vi "Easy2Acquire.IDevice.Acquire.vi"(0 "IDeviceIn":refnum<k7>, 1 "IAnalogInput":refnum<k7>[](array[refnum]), 3 "DigitalInput":refnum<k7>[](array[refnum]), 4 "MotionInput":refnum<k7>[](array[refnum]), 5 "error in (no error)":errorcluster, 6 "stopcapture":refnum<vi>, 7 "AnalgoChart":refnum<vi>, 9 "endprogram":refnum<vi>, 10 "3DRef":refnum<vi>, 11 "DigitalChart":refnum<vi>, 12 "3D Picture":refnum<vi>, 13 "MotionChart":refnum<vi>) -> (14 "AnalogBuffer":dbl[][](array[numeric]), 17 "MotionBuffer":dbl[][][](array[numeric]), 18 "Euler":dbl[][][](array[numeric]), 19 "error out":errorcluster)   [LabVIEW 2017]
panel:
  out "DigitalFrequency":dbl[](array[numeric])
  out "MotionFrequency":dbl[](array[numeric])
  out "DigitalBuffer":i32[][](array[numeric])
  out "ActualFrequency":dbl[](array[numeric])
  in  "stop":bool
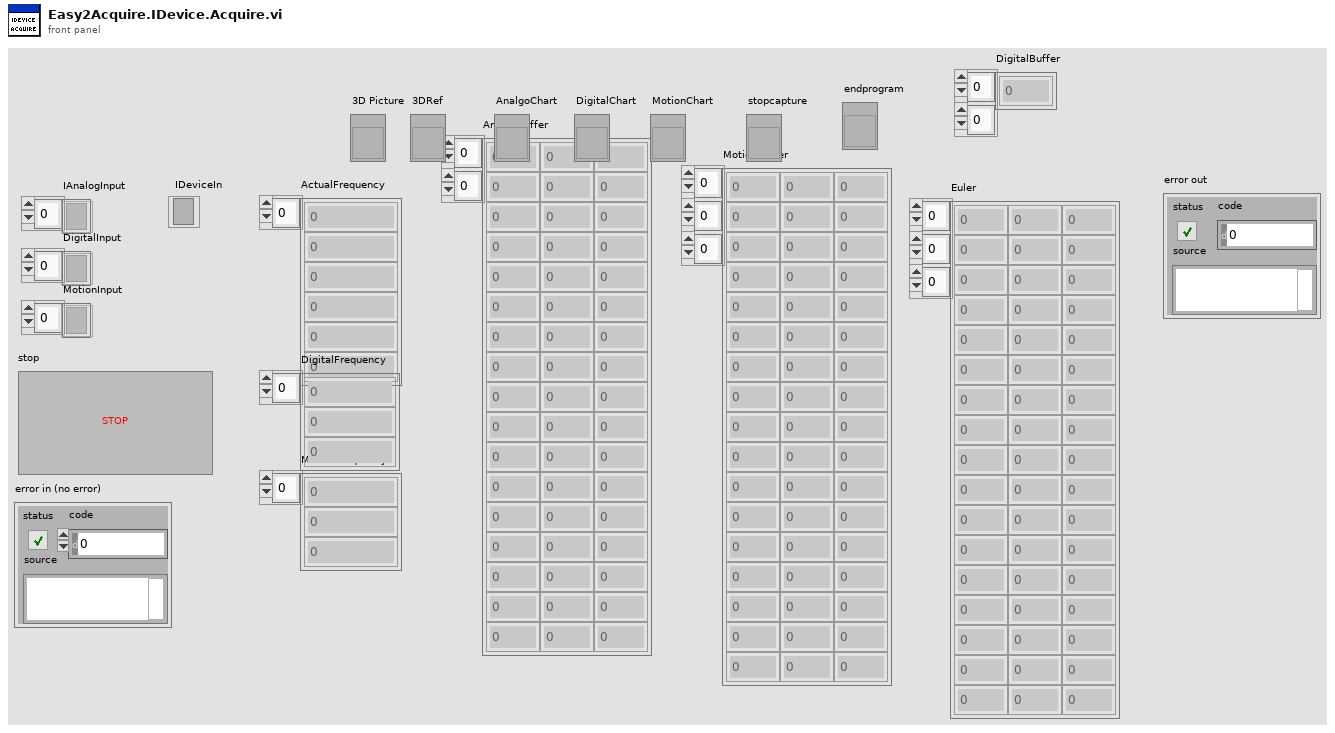
[diagram p1: front panel]
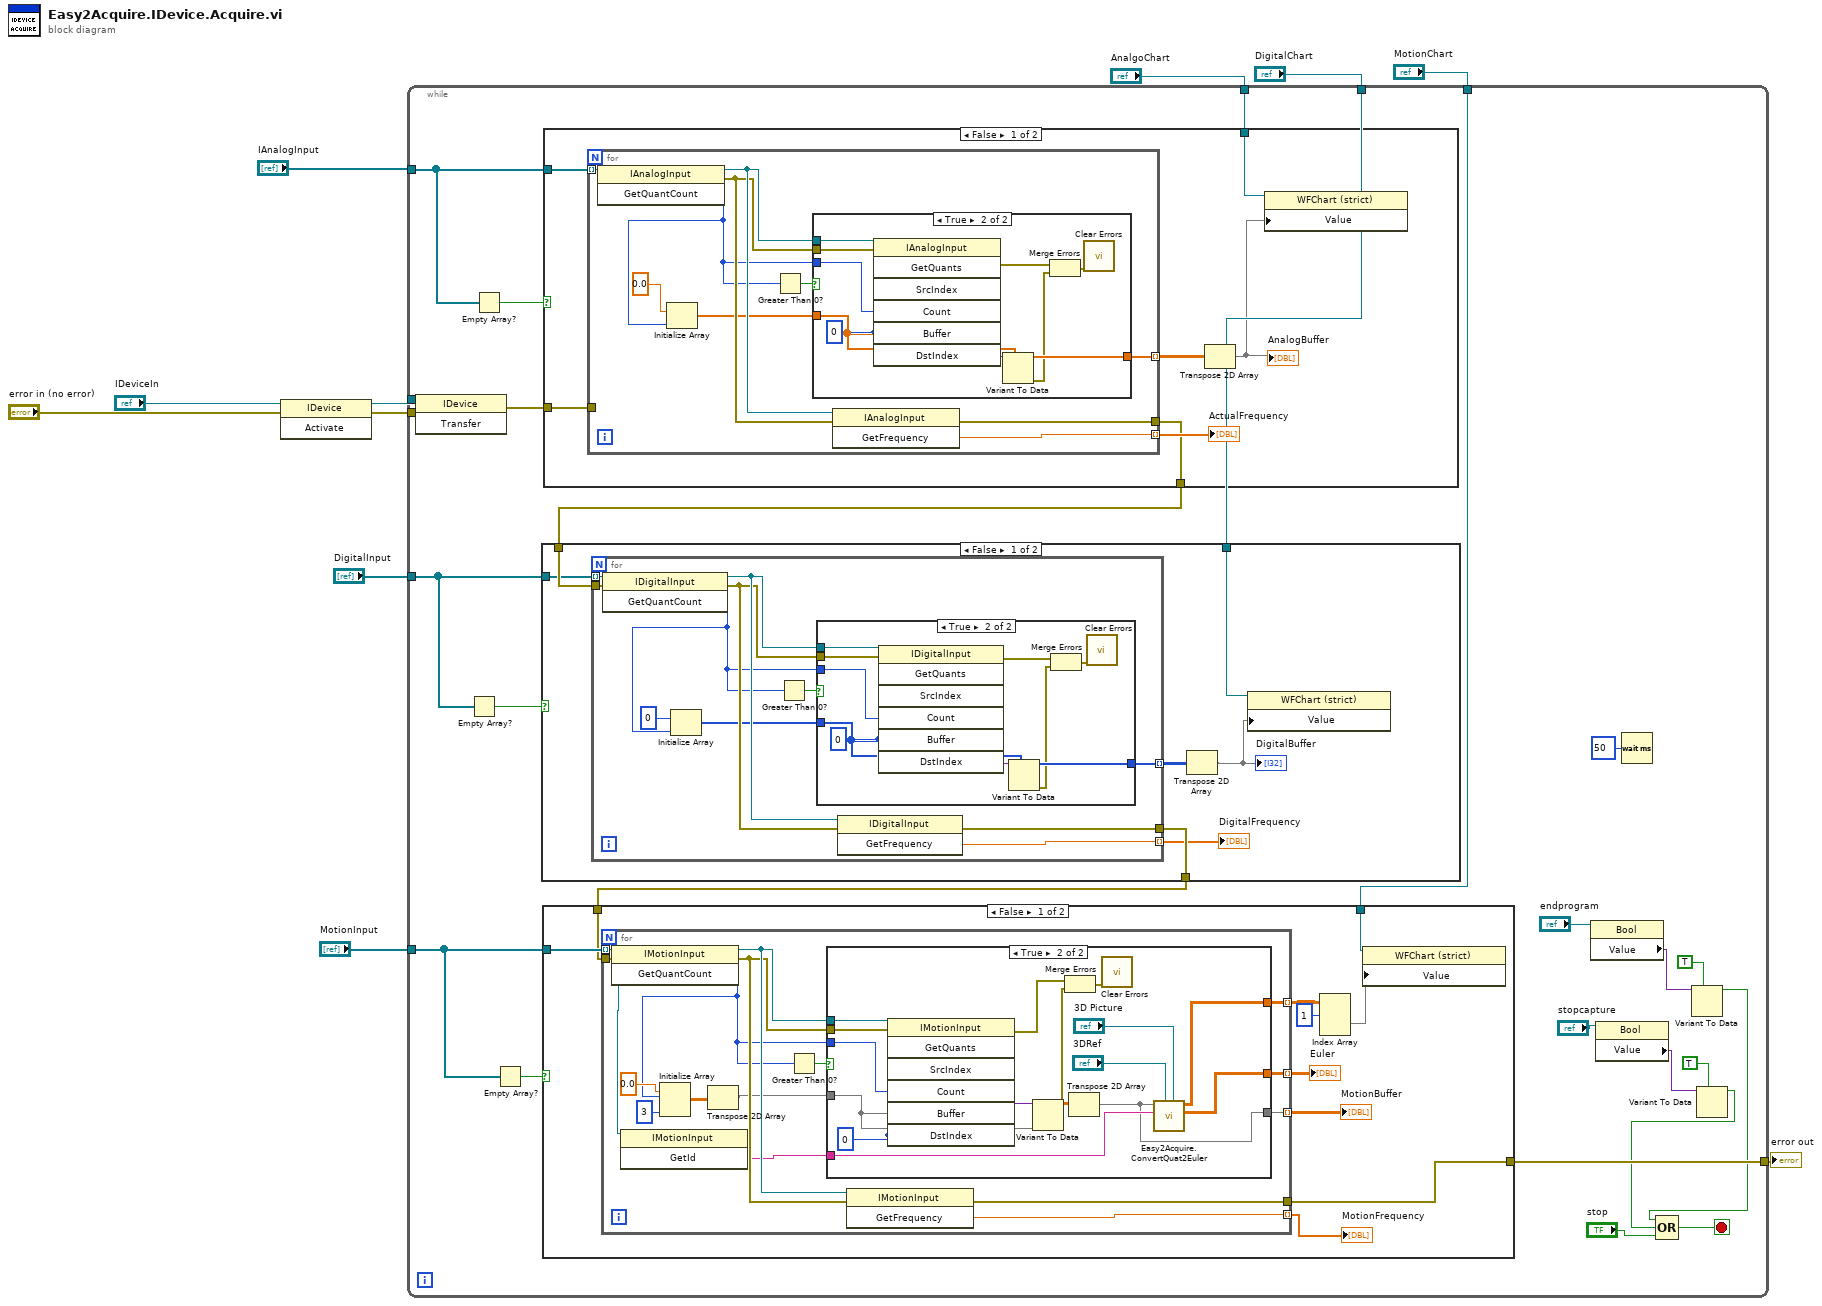
[diagram p0: block diagram]
diagram:
  n1 = invoke class="IDevice" method="Activate"(reference="IDeviceIn", error in="error in (no error)") -> (reference out=w10:refnum<k7>, error out=w9:errorcluster)  [unwired: 1 in, 1 out]
  n2 = while {
    tunnel: "IAnalogInput" -> [w22]
    tunnel: w9 -> [w37]
    tunnel: w10 -> [w36]
    tunnel: "DigitalInput" -> [w20]
    tunnel: "MotionInput" -> [w17]
    tunnel: [w31] -> w4
    tunnel: "AnalgoChart" -> [w30]
    tunnel: "DigitalChart" -> [w23]
    tunnel: "MotionChart" -> [w16]
    stop <- w27 stop-if-true
    n3 = invoke class="IDevice" method="Transfer"(reference=w36, error in=w37) -> (error out=w34:errorcluster)  [unwired: 1 in, 2 out]
    n4 = Empty Array?(array=w20) -> (empty?=w19:bool)
    n5 = Empty Array?(array=w22) -> (empty?=w21:bool)
    n6 = Empty Array?(array=w17) -> (empty?=w18:bool)
    n7 = case shown="False" w21 {
      tunnel: w22 -> [w116 _]
      tunnel: w34 -> [w114 w137]
      tunnel: [w113 w137] -> w33
      tunnel: w30 -> [w112 _]
      frame False {
        n8 = for {
          tunnel: w116 -> [w126] mode=indexing
          tunnel: [w124] -> w115 mode=indexing
          tunnel: [w118] -> w111 mode=indexing
          tunnel: w114 -> [_]
          tunnel: [w117] -> w113
          n9 = invoke class="IAnalogInput" method="GetQuantCount"(reference=w126) -> (reference out=w123:refnum<k7>, error out=w122:errorcluster, "GetQuantCount"=w120:i32)  [unwired: 2 in]
          n10 = Initialize Array(0.0, w120) -> (w121:dbl[])
          n11 = Greater Than 0?(x=w120) -> (x > 0?=w125:bool)
          n12 = case shown="True" w125 {
            tunnel: w123 -> [_ w136]
            tunnel: w120 -> [_ w135]
            tunnel: w122 -> [_ w133]
            tunnel: w121 -> [_ w131]
            tunnel: [_ w130] -> w118
            frame False {
            }
            frame True {
              w134 = 0 ("SrcIndex")
              n13 = invoke class="IAnalogInput" method="GetQuants"(reference=w136, error in=w133, "SrcIndex"=w134, "Count"=w135, "Buffer"=w131, "DstIndex"=w134) -> (error out=w128:errorcluster, "Buffer"=w132:variant)  [unwired: 1 in, 5 out]
              n14 = Variant To Data(type=w131, Variant=w132) -> (data=w130:dbl[], error out=w127:errorcluster)  [unwired: 1 in]
              n15 = Merge Errors(w128, w127) -> (w129:errorcluster)
              n16 = call <vilib>:"Clear Errors.vi"("error in (no error)"=w129) -> ()  [unwired: 5 in, 2 out]
            }
          }
          n17 = invoke class="IAnalogInput" method="GetFrequency"(reference=w123, error in=w122) -> (error out=w117:errorcluster, "GetFrequency"=w124:dbl)  [unwired: 1 in, 1 out]
        }
        "ActualFrequency" <- w115
        n18 = Transpose 2D Array(2D array=w111) -> (transposed array=w110:dbl[][])
        "AnalogBuffer" <- w110
        n19 = property class="WFChart (strict)"(reference=w112, "Value"=w110) -> ()  [unwired: 1 in, 2 out]
      }
      frame True {
      }
    }
    n20 = case shown="False" w19 {
      tunnel: w33 -> [w87 w109]
      tunnel: w20 -> [w86 _]
      tunnel: [w85 w109] -> w32
      tunnel: w23 -> [w82 _]
      frame False {
        n21 = for {
          tunnel: [w97] -> w81 mode=indexing
          tunnel: [w92] -> w84 mode=indexing
          tunnel: w87 -> [w91]
          tunnel: w86 -> [w90] mode=indexing
          tunnel: [w89] -> w85
          n22 = invoke class="IDigitalInput" method="GetQuantCount"(reference=w90, error in=w91) -> (reference out=w96:refnum<k7>, error out=w95:errorcluster, "GetQuantCount"=w93:i32)  [unwired: 1 in]
          n23 = Initialize Array(u8 0, w93) -> (w94:u8[])
          n24 = Greater Than 0?(x=w93) -> (x > 0?=w98:bool)
          n25 = case shown="True" w98 {
            tunnel: w96 -> [_ w108]
            tunnel: w93 -> [_ w107]
            tunnel: w95 -> [_ w105]
            tunnel: w94 -> [_ w103]
            tunnel: [_ w102] -> w92
            frame False {
            }
            frame True {
              w106 = 0 ("SrcIndex")
              n26 = invoke class="IDigitalInput" method="GetQuants"(reference=w108, error in=w105, "SrcIndex"=w106, "Count"=w107, "Buffer"=w103, "DstIndex"=w106) -> (error out=w100:errorcluster, "Buffer"=w104:variant)  [unwired: 1 in, 5 out]
              n27 = Variant To Data(type=w103, Variant=w104) -> (data=w102:u8[], error out=w99:errorcluster)  [unwired: 1 in]
              n28 = Merge Errors(w100, w99) -> (w101:errorcluster)
              n29 = call <vilib>:"Clear Errors.vi"("error in (no error)"=w101) -> ()  [unwired: 5 in, 2 out]
            }
          }
          n30 = invoke class="IDigitalInput" method="GetFrequency"(reference=w96, error in=w95) -> (error out=w89:errorcluster, "GetFrequency"=w97:dbl)  [unwired: 1 in, 1 out]
        }
        "DigitalFrequency" <- w81
        n31 = Transpose 2D Array(2D array=w84) -> (transposed array=w83:u8[][])
        "DigitalBuffer" <- w83
        n32 = property class="WFChart (strict)"(reference=w82, "Value"=w83) -> ()  [unwired: 1 in, 2 out]
      }
      frame True {
      }
    }
    n33 = case shown="False" w18 {
      tunnel: w17 -> [w47 _]
      tunnel: w32 -> [w45 w80]
      tunnel: [w44 w80] -> w31
      tunnel: w16 -> [w42 _]
      frame False {
        n34 = for {
          tunnel: w47 -> [w51] mode=indexing
          tunnel: [w62] -> w43 mode=indexing
          tunnel: [w58] -> w46 mode=indexing
          tunnel: w45 -> [w57]
          tunnel: [w56] -> w44
          tunnel: [w49] -> w41 mode=indexing
          tunnel: [w48] -> w38 mode=indexing
          n35 = invoke class="IMotionInput" method="GetQuantCount"(reference=w51, error in=w57) -> (reference out=w61:refnum<k7>, error out=w60:errorcluster, "GetQuantCount"=w55:i32)  [unwired: 1 in]
          n36 = invoke class="IMotionInput" method="GetId"(reference=w51) -> ("GetId"=w50:string)  [unwired: 2 in, 2 out]
          n37 = Initialize Array(0.0, w55, 3 ("dimension size")) -> (w53:dbl[][])
          n38 = Transpose 2D Array(2D array=w53) -> (transposed array=w52:dbl[][])
          n39 = Greater Than 0?(x=w55) -> (x > 0?=w63:bool)
          n40 = case shown="True" w63 {
            tunnel: w61 -> [_ w79]
            tunnel: w55 -> [_ w78]
            tunnel: w60 -> [_ w76]
            tunnel: w52 -> [_ w74]
            tunnel: [_ w68] -> w58
            tunnel: w50 -> [_ w69]
            tunnel: [_ w67] -> w49
            tunnel: [_ w64] -> w48
            frame False {
            }
            frame True {
              w77 = 0 ("SrcIndex")
              n41 = invoke class="IMotionInput" method="GetQuants"(reference=w79, error in=w76, "SrcIndex"=w77, "Count"=w78, "Buffer"=w74, "DstIndex"=w77) -> (error out=w72:errorcluster, "Buffer"=w75:variant)  [unwired: 1 in, 5 out]
              n42 = Variant To Data(type=w74, Variant=w75) -> (data=w70:dbl[][], error out=w73:errorcluster)  [unwired: 1 in]
              n43 = Merge Errors(w72, w73) -> (w71:errorcluster)
              n44 = Transpose 2D Array(2D array=w70) -> (transposed array=w68:dbl[][])
              n45 = call <vilib>:"Clear Errors.vi"("error in (no error)"=w71) -> ()  [unwired: 5 in, 2 out]
              n46 = call "Easy2Acquire.ConvertQuat2Euler.vi"("3D Picture"="3D Picture", "3DRef"="3DRef", "GetID"=w69, "MotionData"=w68) -> ("Euler"=w64:dbl[][], "Accel"=w67:dbl[][])  [unwired: 6 in]
            }
          }
          n47 = invoke class="IMotionInput" method="GetFrequency"(reference=w61, error in=w60) -> (error out=w56:errorcluster, "GetFrequency"=w62:dbl)  [unwired: 1 in, 1 out]
        }
        "MotionBuffer" <- w46
        "MotionFrequency" <- w43
        "Euler" <- w38
        n48 = Index Array(array=w41, index (dim 0)=1 ("index (page)")) -> (element=w40:dbl[][])  [unwired: 2 in]
        n49 = property class="WFChart (strict)"(reference=w42, "Value"=w40) -> ()  [unwired: 1 in, 2 out]
      }
      frame True {
      }
    }
    n50 = property class="Bool"(reference="endprogram") -> ("Value"=w15:variant)  [unwired: 1 in, 2 out]
    n51 = property class="Bool"(reference="stopcapture") -> ("Value"=w26:variant)  [unwired: 1 in, 2 out]
    n52 = Wait (ms)(milliseconds to wait=u32 50) -> ()  [unwired: 1 out]
    n53 = Variant To Data(type=TRUE, Variant=w15) -> (data=w12:bool)  [unwired: 1 in, 1 out]
    n54 = Variant To Data(type=TRUE, Variant=w26) -> (data=w24:bool)  [unwired: 1 in, 1 out]
    n55 = Compound Arithmetic op=OR(w12, w24, "stop") -> (w27:bool)
  }
  "error out" <- w4
